vi "Unlock ECU.vi"(8 "error in (no error)":errorcluster, 11 "Node Ptr":T2 format="%.0x") -> (0 "error out":errorcluster)   [LabVIEW 2019, in "Diagnostics Addon System Explorer.lvlib"]
uses:
  Diagnostics Addon System Explorer.lvlib
  Addon Shared/Types/Security.Type.ctl
  <vilib>/NI VeriStand/Custom Device API/Custom Device Item Ref.ctl
  Types/FG.Action.ctl
  Addon Shared/Types/Settings.Channel.ctl
  <vilib>/NI VeriStand/Custom Device API/Custom Device Channel.ctl
  <vilib>/NI VeriStand/Custom Device API/Custom Device Channel Type.ctl
  SubVIs/FileDependency.Create.vi
  Addon Shared/SubVIs/Constants.vi
  SubVIs/FileDependency.Get.Target Path.vi
  <vilib>/NI VeriStand/Custom Device API/NI VeriStand - Get Item Property.vi
  <vilib>/NI VeriStand/Custom Device API/Get Item Property (U32).vi
  <vilib>/Utility/MD5Checksum.llb/MD5Checksum File.vi
  <vilib>/NI/NI VeriStand Advanced SysDef API/SysDef API/SysDef.Property.Set.vi
  <vilib>/NI/NI VeriStand Advanced SysDef API/_SubVIs/SysDef.Property.Set.DependentFile.vi
  <vilib>/NI/NI VeriStand Advanced SysDef API/SysDef API/SysDef.Property.Remove.vi
  <vilib>/NI/NI VeriStand Advanced SysDef API/_SubVIs/SysDef.Property.Set.U32.vi
  <vilib>/NI VeriStand/Custom Device Tools/Custom Device Utility Library/NI VeriStand - Search for Item by GUID.vi
  <vilib>/NI VeriStand/Custom Device API/Custom Device API.lvlib
  Addon Shared/Diagnostics Addon Shared.lvlib
  <vilib>/NI VeriStand/Custom Device Tools/Custom Device Utility Library/Custom Device Utility Library.lvlib
panel:
  in  "Access Mode":u8 format="%.0x"
  in  "Seed Key Path":path caption="Seed Key Path (.DLL or .SO)"
  in  "Type":T1
  in  "Master Key":string
  in  "Header":cluster{"Section Name":string}={"Section Name"="Security Settings"}
  in  "SHDocVw.IWebBrowser":refnum<k7>(container)
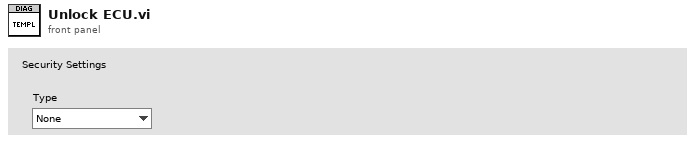
[diagram p1: front panel]
types:
  T1 = typedef "Diagnostics Addon Shared.lvlib/Security.Type.ctl" = enum16{"None", "SeedKey", "MasterKey"}
  T2 = typedef "Custom Device API.lvlib/Custom Device Item Ref.ctl" = u64
  T3 = typedef "Diagnostics Addon System Explorer.lvlib/FG.Action.ctl" = enum16{"Get", "Set"}
  T4 = typedef "Custom Device API.lvlib/Custom Device Item Info.ctl" = cluster{"Name":string, "Is Channel":bool, "GUID":string, "Is Waveform":bool}
  T5 = typedef "Diagnostics Addon Shared.lvlib/Security.ctl" = cluster{"Type":T1, "Source DLL Path":path, "Target DLL Path":path, "Security Level":u8}
  T6 = typedef "Custom Device API.lvlib/Custom Device Commands.ctl" = enum16{"Default", "Item renamed", "Shutdown", "Dynamic button pressed"}
  T7 = typedef "Diagnostics Addon Shared.lvlib/Settings.Channel.ctl" = cluster{"Name":string, "Description":string, "Channel":T8}
  T8 = typedef "Custom Device API.lvlib/Custom Device Channel.ctl" = cluster{"Type":T9, "Units":string, "Default Value":dbl, "Faultable":bool, "Scalable":bool}
  T9 = typedef "Custom Device API.lvlib/Custom Device Channel Type.ctl" = enum16{"Input", "Output"}
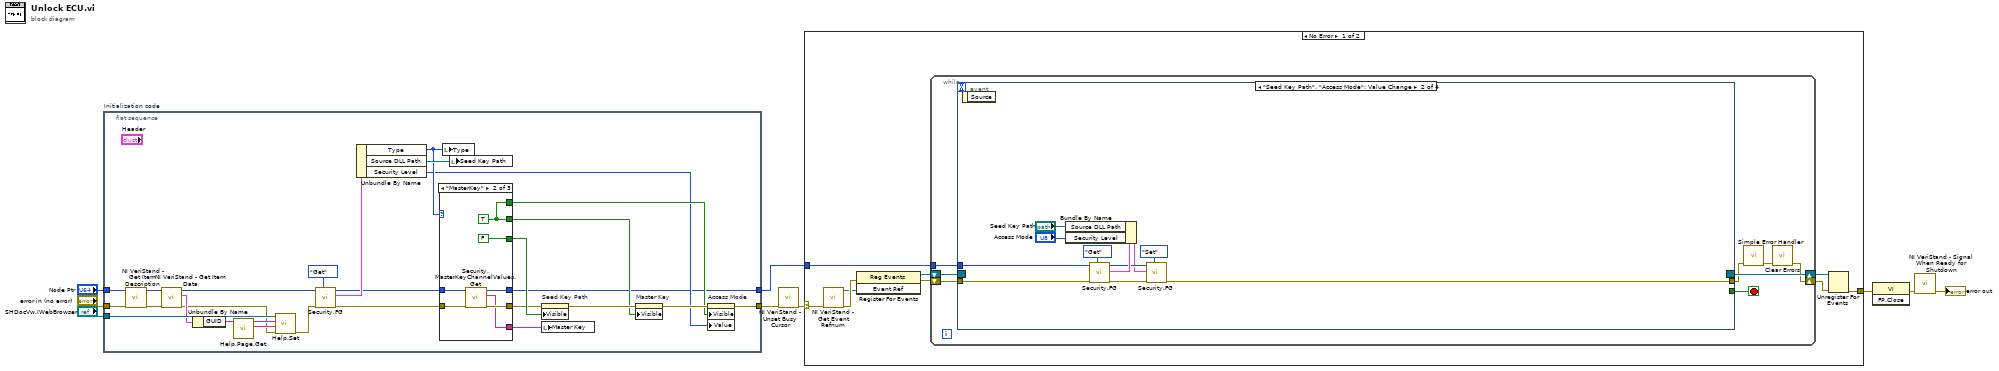
[diagram p0: block diagram]
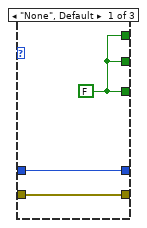
[diagram p2: hidden frame]
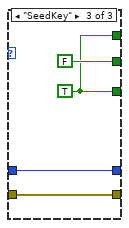
[diagram p3: hidden frame]
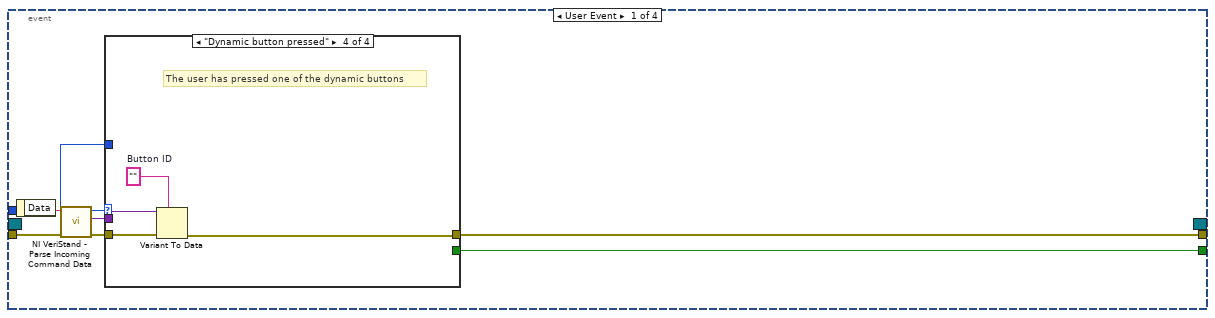
[diagram p4: hidden frame]
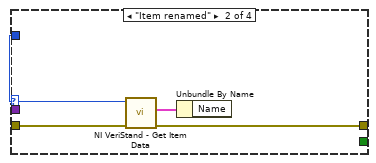
[diagram p6: hidden frame]
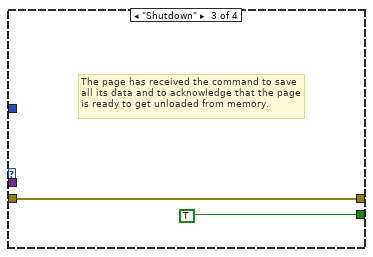
[diagram p7: hidden frame]
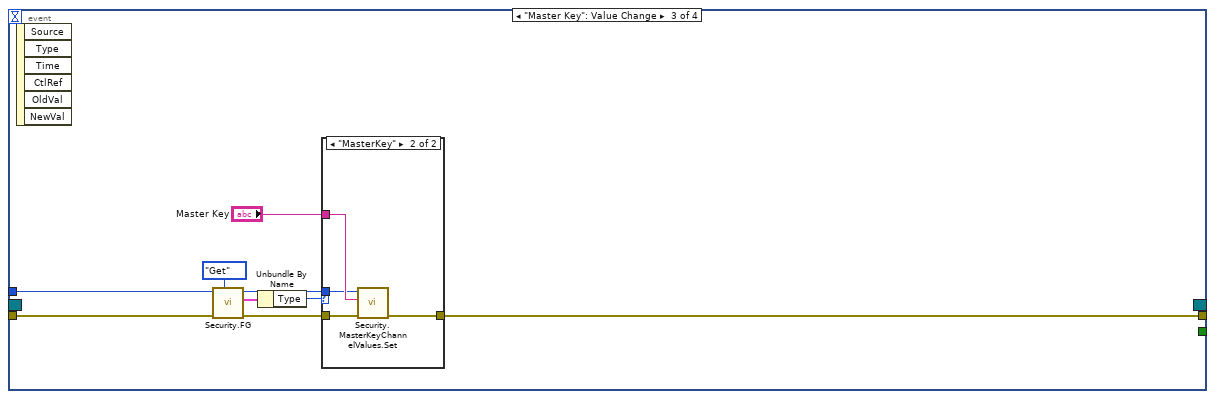
[diagram p8: hidden frame]
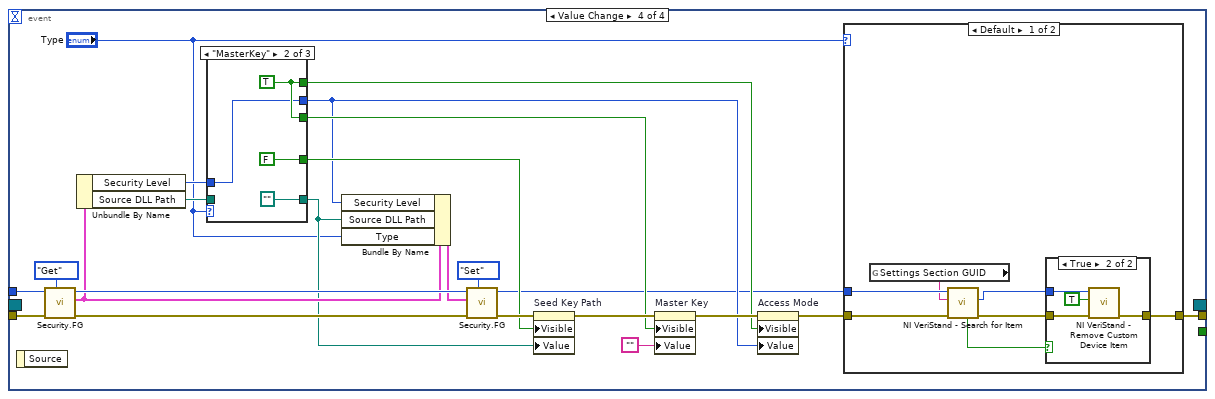
[diagram p10: hidden frame]
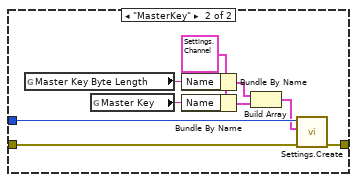
[diagram p12: hidden frame]
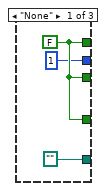
[diagram p13: hidden frame]
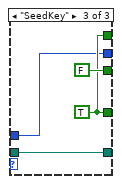
[diagram p14: hidden frame]
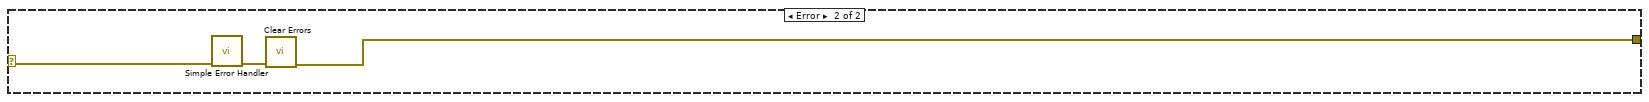
[diagram p15: hidden frame]
diagram:
  n1 = flat-sequence "Initialization code" {
    tunnel: "error in (no error)" -> [w19]
    tunnel: "Node Ptr" -> [w22]
    tunnel: [w26] -> w5
    tunnel: [w11] -> w2
    tunnel: "SHDocVw.IWebBrowser" -> [w35]
    frame #0 {
      n2 = call <vilib>:"NI VeriStand - Get Item Description.vi"("error in (no error)"=w19, "Item Ref in"=w22) -> ("error out"=w36:errorcluster, "Item Ref out"=w37:T2)  [unwired: 8 out]
      n3 = call <vilib>:"NI VeriStand - Get Item Data.vi"("error in (no error)"=w36, "Item Ref in"=w37) -> ("error out"=w16:errorcluster, "Item Info"=w18:T4, "Item Ref out"=w23:T2)  [unwired: 7 out]
      n4 = Unbundle By Name(w18) -> ("GUID"=w17:string)
      n5 = call "Help.Page.Get.vi"("GUID"=w17) -> ("HTML File"=w20:string, "Main CHM File"=w21:string)  [unwired: 9 in]
      n6 = call "Help.Set.vi"("error in (no error)"=w16, "HTML File"=w20, "Main CHM File"=w21, "SHDocVw.IWebBrowser2"=w35) -> ("error out"=w15:errorcluster)  [unwired: 7 in]
      n7 = call "Security.FG.vi"("Action"=FG.Action."Get", "error in (no error)"=w15, "Device Item Ref in"=w23) -> ("error out"=w13:errorcluster, "Security"=w34:T5, "Device Item Ref out"=w14:T2)  [unwired: 6 in]
      n8 = Unbundle By Name(w34) -> ("Type"=w30:T1, "Source DLL Path"=w32:path, "Security Level"=w24:u8)
      n9 = case shown="\"MasterKey\"" w30 {
        tunnel: [w40 FALSE w50] -> w29
        tunnel: [w40 w46 FALSE] -> w28
        tunnel: [w40 w46 w50] -> w25
        tunnel: w14 -> [w38 w44 w48]
        tunnel: w13 -> [w39 w45 w49]
        tunnel: [w39 w43 w49] -> w12
        tunnel: [w38 w42 w48] -> w11
        tunnel: [_ w41 _] -> w10
        frame "None", Default {
          w40 = FALSE
        }
        frame "MasterKey" {
          w46 = TRUE
          n10 = call "Security.MasterKeyChannelValues.Get.vi"("error in (no error)"=w45, "Device Item Ref in"=w44) -> ("error out"=w43:errorcluster, "MasterKey"=w41:string, "Section Ref out"=w42:T2)  [unwired: 7 in]
        }
        frame "SeedKey" {
          w50 = TRUE
        }
      }
      n11 = local write "Type"(w30) -> ()
      n12 = local write "Seed Key Path"(w32) -> ()
      n13 = property on="Seed Key Path" class="Path"(error in=w12, "Visible"=w29) -> (error out=w31:errorcluster)  [unwired: 1 in, 1 out]
      n14 = local write "Master Key"(w10) -> ()
      n15 = property on="Master Key" class="Str"(error in=w31, "Visible"=w28) -> (error out=w27:errorcluster)  [unwired: 1 in, 1 out]
      n16 = property on="Access Mode" class="DigNum (strict)"(error in=w27, "Visible"=w25, "Value"=w24) -> (error out=w26:errorcluster)  [unwired: 1 in, 1 out]
    }
  }
  n17 = call <vilib>:"NI VeriStand - Unset Busy Cursor.vi"("error in (no error)"=w5) -> ("error out"=w4:errorcluster)  [unwired: 10 out]
  n18 = case shown="No Error" w4 {
    selector: w4 -> [w52 w170]
    tunnel: [w57 w168] -> w9
    tunnel: w2 -> [w53 _]
    frame No Error {
      n19 = call <vilib>:"NI VeriStand - Get Event Refnum.vi"("error in (no error)"=w52) -> ("error out"=w60:errorcluster, "Event Ref"=w56:refnum<user-event>)  [unwired: 9 out]
      n20 = register-events(error in=w60, w56) -> (reference out=w54:refnum<event-registration>, error out=w55:errorcluster)  [unwired: 1 in]
      n21 = while {
        tunnel: w53 -> [w64]
        shift-right: [w61] -> w58
        shift-left: w55 -> [w67]
        shift-right: [w68] -> w59
        shift-left: w54 -> [w66]
        stop <- w65 stop-if-true
        n22 = event shown="[1] \"Seed Key Path\", \"Access Mode\": Value Change" {
          selector: w66 -> [_ _ _ _]
          dyn-events: [_ _ _ _] -> w68
          timeout: _ -> [_ _ _ _]
          tunnel: w67 -> [w76 w98 w107 w135]
          tunnel: [w72 _ _ _] -> w65
          tunnel: [w71 w88 w104 w117] -> w63
          tunnel: w64 -> [w70 w97 w106 w134]
          event User Event {
            n23 = event-data() -> ("Data"=w75:string)  [unwired: 1 out]
            n24 = call <vilib>:"NI VeriStand - Parse Incoming Command Data.vi"("error in (no error)"=w76, "Incoming data"=w75) -> ("error out"=w74:errorcluster, "Outgoing data"=w69:variant, "Action"=w73:T6)  [unwired: 7 out]
            n25 = case shown="\"Dynamic button pressed\"" w73 {
              tunnel: w74 -> [w77 w81 w82 w87]
              tunnel: [_ _ TRUE _] -> w72
              tunnel: [w77 w78 w82 w84] -> w71
              tunnel: w70 -> [_ w80 _ _]
              tunnel: w69 -> [_ _ _ w86]
              frame "Default", Default {
              }
              frame "Item renamed" {
                n26 = call <vilib>:"NI VeriStand - Get Item Data.vi"("error in (no error)"=w81, "Item Ref in"=w80) -> ("error out"=w78:errorcluster, "Item Info"=w79:T4)  [unwired: 8 out]
                n27 = Unbundle By Name(w79) -> ()  [unwired: 1 out]
              }
              frame "Shutdown" {
                # "The page has received the command to save all its data and to acknowledge that the page is ready to get unloaded from memory."
              }
              frame "Dynamic button pressed" {
                w85 = ""  # Button ID
                # "The user has pressed one of the dynamic buttons"
                n28 = Variant To Data(error in=w87, type=w85, Variant=w86) -> (error out=w84:errorcluster)  [unwired: 1 out]
              }
            }
          }
          event "Seed Key Path", "Access Mode": Value Change {
            n29 = event-data() -> ()  [unwired: 2 out]
            n30 = call "Security.FG.vi"("Action"=FG.Action."Get", "error in (no error)"=w98, "Device Item Ref in"=w97) -> ("error out"=w94:errorcluster, "Security"=w96:T5, "Device Item Ref out"=w93:T2)  [unwired: 6 in]
            n31 = Bundle By Name(cluster=w96, "Source DLL Path"="Seed Key Path", "Security Level"="Access Mode") -> (w89:T5)
            n32 = call "Security.FG.vi"("Action"=FG.Action."Set", "error in (no error)"=w94, "Security"=w89, "Device Item Ref in"=w93) -> ("error out"=w88:errorcluster)  [unwired: 5 in, 2 out]
          }
          event "Master Key": Value Change {
            n33 = event-data() -> ()  [unwired: 7 out]
            n34 = call "Security.FG.vi"("Action"=FG.Action."Get", "error in (no error)"=w107, "Device Item Ref in"=w106) -> ("error out"=w103:errorcluster, "Security"=w101:T5, "Device Item Ref out"=w102:T2)  [unwired: 6 in]
            n35 = Unbundle By Name(w101) -> ("Type"=w99:T1)
            n36 = case shown="\"MasterKey\"" w99 {
              tunnel: [w108 w111] -> w104
              tunnel: w103 -> [w108 w112]
              tunnel: "Master Key" -> [_ w110]
              tunnel: w102 -> [_ w109]
              frame Default {
              }
              frame "MasterKey" {
                n37 = call "Security.MasterKeyChannelValues.Set.vi"("error in (no error)"=w112, "Master Key"=w110, "Device Item Ref in"=w109) -> ("error out"=w111:errorcluster)  [unwired: 7 in, 1 out]
              }
            }
          }
          event Value Change {
            n38 = event-data() -> ()  [unwired: 2 out]
            n39 = call "Security.FG.vi"("Action"=FG.Action."Get", "error in (no error)"=w135, "Device Item Ref in"=w134) -> ("error out"=w132:errorcluster, "Security"=w124:T5, "Device Item Ref out"=w131:T2)  [unwired: 6 in]
            n40 = Unbundle By Name(w124) -> ("Security Level"=w119:u8, "Source DLL Path"=w123:path)
            n41 = case shown="\"MasterKey\"" "Type" {
              tunnel: [w158 FALSE w165] -> w126
              tunnel: [w158 w161 FALSE] -> w125
              tunnel: w123 -> [_ _ w166]
              tunnel: [path "" path "" w166] -> w122
              tunnel: [w158 w161 w165] -> w120
              tunnel: w119 -> [_ w160 w164]
              tunnel: [u8 1 w160 w164] -> w116
              frame "None" {
                w158 = FALSE
              }
              frame "MasterKey" {
                w161 = TRUE
              }
              frame "SeedKey" {
                w165 = TRUE
              }
            }
            n42 = Bundle By Name(cluster=w124, "Security Level"=w116, "Source DLL Path"=w122, "Type"="Type") -> (w129:T5)
            n43 = call "Security.FG.vi"("Action"=FG.Action."Set", "error in (no error)"=w132, "Security"=w129, "Device Item Ref in"=w131) -> ("error out"=w127:errorcluster, "Device Item Ref out"=w114:T2)  [unwired: 5 in, 1 out]
            n44 = property on="Seed Key Path" class="Path"(error in=w127, "Visible"=w126, "Value"=w122) -> (error out=w128:errorcluster)  [unwired: 1 in, 1 out]
            n45 = property on="Master Key" class="Str"(error in=w128, "Visible"=w125, "Value"="") -> (error out=w121:errorcluster)  [unwired: 1 in, 1 out]
            n46 = property on="Access Mode" class="DigNum (strict)"(error in=w121, "Visible"=w120, "Value"=w116) -> (error out=w118:errorcluster)  [unwired: 1 in, 1 out]
            n47 = case shown="Default" "Type" {
              tunnel: w118 -> [w140 w156]
              tunnel: [w141 w155] -> w117
              tunnel: w114 -> [w142 w154]
              frame Default {
                n48 = global read "Constants.vi" "Settings Section GUID"() -> (w137:string)
                n49 = call-poly <vilib>:"NI VeriStand - Search for Item.vi"("error in"=w140, "Item GUID"=w137, "Section Ref in"=w142) -> ("error out"=w139:errorcluster, "Item Ref"=w138:T2, "Found"=w136:bool)  [unwired: 5 in, 1 out]
                n50 = case shown="True" w136 {
                  tunnel: [w143 w147] -> w141
                  tunnel: w139 -> [w143 w146]
                  tunnel: w138 -> [_ w145]
                  frame False {
                  }
                  frame True {
                    n51 = call <vilib>:"NI VeriStand - Remove Custom Device Item.vi"("error in (no error)"=w146, "Force Delete (F)"=TRUE, "Item Ref in"=w145) -> ("error out"=w147:errorcluster)  [unwired: 7 in, 1 out]
                  }
                }
              }
              frame "MasterKey" {
                w148 = T7 {"Name"="Byte Length", "Description"="", "Channel"={"Type"=enum."Input", "Units"="", "Default Value"=0.0, "Faultable"=FALSE, "Scalable"=FALSE}} ("cluster")
                n52 = global read "Constants.vi" "Master Key Byte Length"() -> (w150:string)
                n53 = global read "Constants.vi" "Master Key"() -> (w149:string)
                n54 = Bundle By Name(cluster=w148, "Name"=w150) -> (w151:T7)
                n55 = Bundle By Name(cluster=w148, "Name"=w149) -> (w153:T7)
                n56 = Build Array(w151, w153) -> (w152:T7[])
                n57 = call "Settings.Create.vi"("error in (no error)"=w156, "Settings Channels"=w152, "Section Ref in"=w154) -> ("error out"=w155:errorcluster)  [unwired: 7 in, 1 out]
              }
            }
          }
        }
        n58 = call <vilib>:"Simple Error Handler.vi"("error in (no error)"=w63) -> ("error out"=w62:errorcluster)  [unwired: 1 in, 7 out]
        n59 = call <vilib>:"Clear Errors.vi"("error in (no error)"=w62) -> ("error out"=w61:errorcluster)  [unwired: 1 in, 5 out]
      }
      n60 = Unregister For Events(event registration refnum=w59, error in=w58) -> (error out=w57:errorcluster)
    }
    frame Error {
      n61 = call <vilib>:"Simple Error Handler.vi"("error in (no error)"=w170) -> ("error out"=w169:errorcluster)  [unwired: 1 in, 7 out]
      n62 = call <vilib>:"Clear Errors.vi"("error in (no error)"=w169) -> ("error out"=w168:errorcluster)  [unwired: 1 in, 5 out]
    }
  }
  n63 = invoke class="VI" method="FP.Close"(error in=w9) -> (error out=w8:errorcluster)  [unwired: 2 in, 2 out]
  n64 = call <vilib>:"NI VeriStand - Signal When Ready for Shutdown.vi"("error in (no error)"=w8) -> ("error out"=→"error out":errorcluster)  [unwired: 10 out]
